vi "Update FIFO Empty Flag - 16-bit Address.vi"(0 "empty in":bool, 5 "full count":u16, 7 "write":bool, 9 "read":bool) -> (4 "empty out":bool)   [LabVIEW 2011, in "FIFO.lvlib"]
uses:
  <instrlib>/RF-RIO/FIFO/FIFO/FPGA/FIFO.lvlib
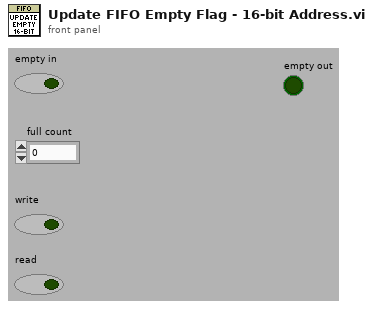
[diagram p1: front panel]
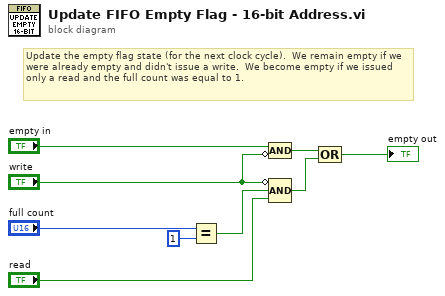
[diagram p0: block diagram]
diagram:
  # "Update the empty flag state (for the next clock cycle).  We remain empty if we were already empty and didn't issue a write.  We become empty if we issued only a read and the full count was equal to 1."
  n1 = Equal?(x="full count", y=u16 1) -> (x = y?=w9:bool)
  n2 = Compound Arithmetic op=AND("empty in", invert "write") -> (w8:bool)
  n3 = Compound Arithmetic op=AND(invert "write", w9, "read") -> (w7:bool)
  n4 = Compound Arithmetic op=OR(w8, w7) -> (→"empty out":bool)
